vi "get_prefix.vi"(8 "error in (no error)":errorcluster, 11 "self in":refnum<class "Identifier.lvclass">) -> (0 "error out":errorcluster, 2 "_prefix_":string, 3 "self out":refnum<class "Identifier.lvclass">)   [LabVIEW 2020, in "mlir.lvlib" / "Identifier.lvclass"]
uses:
  Identifier.lvclass
  Identifier.lvclass/Identifier.ctl
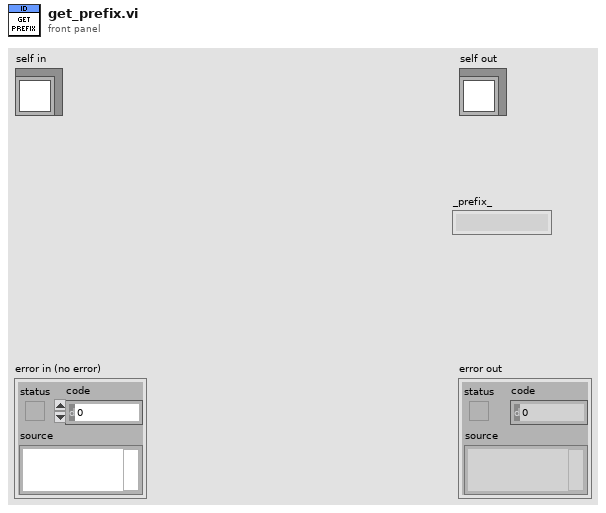
[diagram p1: front panel]
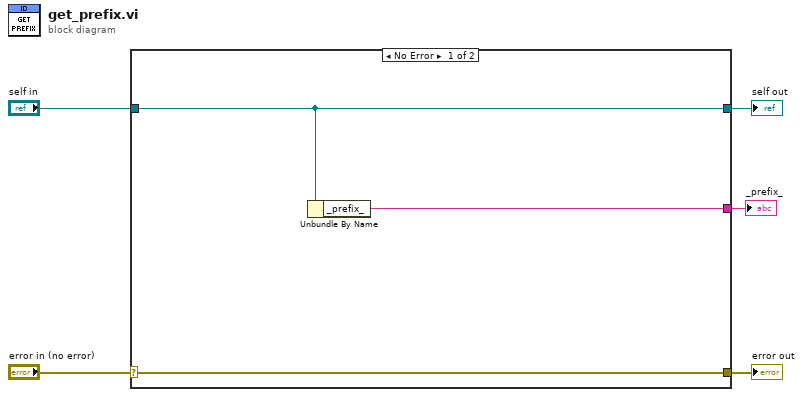
[diagram p0: block diagram]
diagram:
  n1 = case shown="No Error" "error in (no error)" {
    selector: "error in (no error)" -> [w8 w10]
    tunnel: [w8 w10] -> w4
    tunnel: [w7 w9] -> w2
    tunnel: "self in" -> [w7 w9]
    tunnel: [w6 _] -> w1
    frame No Error {
      n2 = Unbundle By Name(w7) -> ("_prefix_"=w6:string)
    }
    frame Error {
    }
  }
  "error out" <- w4
  "self out" <- w2
  "_prefix_" <- w1
